vi "train_conVAE.vi"(0 "error in (no error)":errorcluster, 1 "X":sgl[][](array[numeric]), 2 "X_HAT":sgl[][](array[numeric]), 3 "eta_vae":sgl, 5 "ptr_encoder":i64, 7 "ptr_decoder":i64, 8 "handoverlayer":u32, 9 "ptr_forward":i64, 10 "spec_norm_forw":bool, 11 "eta_forw":sgl, 12 "Y":sgl[][](array[numeric]), 13 "Y_back":sgl[][](array[numeric]), 14 "batch_update":u32, 15 "weight_norm_vae":bool) -> (4 "error out":errorcluster, 6 "error":sgl)   [LabVIEW 2016, in "CNet.lvlib"]
uses:
  CNet.lvlib
  Users/jg754/Documents/Visual Studio 2015/Projects/CLearn/x64/Release/CLearn.dll
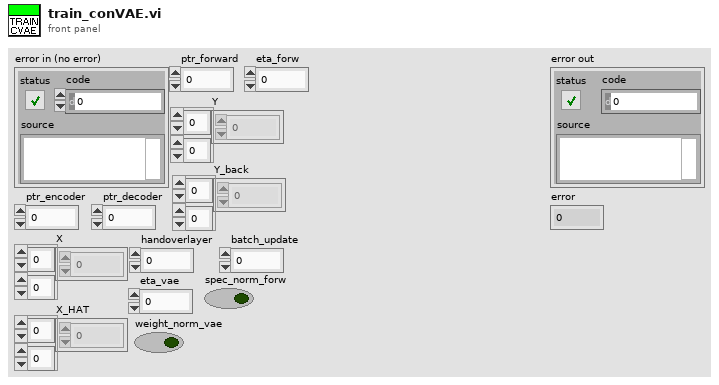
[diagram p1: front panel]
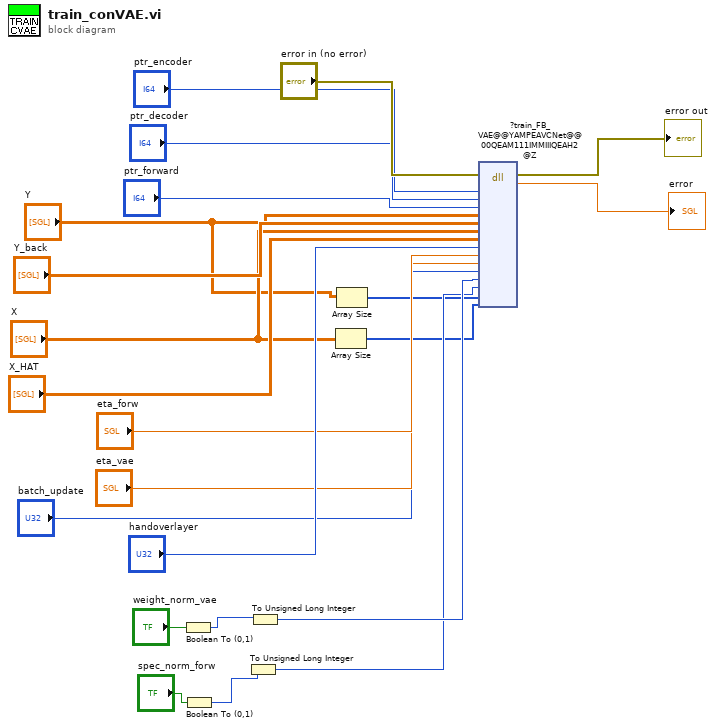
[diagram p0: block diagram]
diagram:
  n1 = Boolean To (0,1)(Boolean="weight_norm_vae") -> (0, 1=w9:i16)
  n2 = Boolean To (0,1)(Boolean="spec_norm_forw") -> (0, 1=w8:i16)
  n3 = To Unsigned Long Integer(number=w8) -> (unsigned 32bit integer=w6:u32)
  n4 = To Unsigned Long Integer(number=w9) -> (unsigned 32bit integer=w7:u32)
  n5 = Array Size(array="X") -> (size(s)=w4:i32[])
  n6 = Array Size(array="Y") -> (size(s)=w2:i32[])
  n7 = dll-call lib="C:/Users/jg754/Documents/Visual Studio 2015/Projects/CLearn/x64/Release/CLearn.dll" fn="?train_FB_VAE@@YAMPEAVCNet@@00QEAM111IMMIIIQEAH2@Z"(error in="error in (no error)", "ptr_encoder"="ptr_encoder", "ptr_decoder"="ptr_decoder", "ptr_forward"="ptr_forward", "Y"="Y", "Y_back"="Y_back", "X"="X", "X_HAT"="X_HAT", "handoverlayer"="handoverlayer", "eta_forw"="eta_forw", "eta_vae"="eta_vae", "batch_update"="batch_update", "weight_norm"=w7, "spectral_norm"=w6, "Y_format"=w2, "X_format"=w4) -> (error out=→"error out":errorcluster, "error"=→"error":sgl)  [unwired: 17 in, 1 out]
